vi "BCU参数读取-Auto.vi"(8 "CAN端口":u16(ring), 9 "设备索引号":u16(ring), 10 "CAN卡类型":u32(ring)=21, 11 "Myindex":dbl=1.0) -> (3 "成功":bool)   [LabVIEW 2013] (continued)
              n1586 = call <vilib>:"Unset Busy.vi"() -> ()  [unwired: 2 in, 10 out]
            }
          }
        }
        frame "模块软件版本读取" {
          n1587 = local read "从板板号"() -> (w2581:u8)
          n1588 = local read "模块软件版本"() -> (w2582:T1)
          n1589 = case shown="\"全部读取\"" w2582 {
            selector: w2582 -> [w2583 w2627]
            tunnel: w2581 -> [_ w2626]
            frame "BCUMCAL", Default {
              n1590 = stacked-sequence {
                seq-local: [_ _ w2609 _] -> [_ _ _ w2616]
                tunnel: w2583 -> [_ w2589 _ w2617]
                frame #0 {
                  w2588 = FALSE ("写?")
                  n1591 = call <vilib>:"Set Busy.vi"("disable click? (T)"=FALSE) -> ()  [unwired: 3 in, 8 out]
                  n1592 = local write "写?"(w2588) -> ()
                  n1593 = global write "EV05全局变量1.vi" "流控帧 2"(TRUE ("流控帧 2")) -> ()
                  n1594 = global write "EV05全局变量1.vi" "写入超时"(w2588) -> ()
                  n1595 = local write "控制1"(TRUE ("控制1")) -> ()
                  n1596 = local write "消除"(TRUE ("消除")) -> ()
                }
                frame #1 {
                  n1597 = Quotient & Remainder(x=w2589, y=256) -> (x-y*floor(x/y)=w2590:i32, floor(x/y)=w2591:i32)
                  n1598 = Build Array(w2591, w2590, u8 0 ("板号")) -> (w2594:i32[])
                  n1599 = local read "设备索引号"() -> (w2596:u16)
                  n1600 = local read "CAN卡类型"() -> (w2597:u32)
                  n1601 = local read "CAN端口"() -> (w2595:u16)
                  n1602 = stacked-sequence {
                    tunnel: w2597 -> [w2600 w2608]
                    tunnel: w2596 -> [w2599 w2607]
                    tunnel: w2595 -> [w2598 w2606]
                    tunnel: w2594 -> [_ w2605]
                    frame #0 {
                      n1603 = dll-call lib="PTH1abs FBluewave New EnergySVN_WorkAutoTest_TestStandtrunkAutoTest_TestStandDriverZlgCanBHN01è¯»ååæ°data\nkerneldlls\nusbcan.dll" fn="VCI_ClearBuffer"("DeviceType"=w2600, "DeviceInd"=w2599, "CANInd"=w2598) -> (error out=w2601:errorcluster)  [unwired: 4 in, 4 out]
                      n1604 = call <vilib>:"Clear Errors.vi"("error in (no error)"=w2601) -> ()  [unwired: 6 in, 1 out]
                    }
                    frame #1 {
                      w2604 = u8 137 ("命令")
                      w2602 = u32 3 ("命令序号")
                      n1605 = local read "从板板号"() -> (w2603:u8)
                      n1606 = local write "命令"(w2604) -> ()
                      n1607 = call "多帧发送机制(EV05).vi"("can卡类型"=w2608, "设备索引号"=w2607, "CAN端口"=w2606, "命令"=w2604, "板号"=w2603, "命令序号"=w2602, "输入数据"=w2605) -> ()  [unwired: 2 in, 11 out]
                      n1608 = local write "命令序号"(w2602) -> ()
                    }
                  }
                }
                frame #2 {
                  n1609 = while {
                    tunnel: [w2610] -> w2609
                    i -> [w2615]
                    stop <- w2611 stop-if-true
                    n1610 = global read "EV05全局变量1.vi" "写入超时"() -> (w2610:bool)
                    n1611 = Greater Or Equal?(x=w2615, y=25) -> (x >= y?=w2612:bool)
                    n1612 = Or(x=w2610, y=w2612) -> (x .or. y?=w2611:bool)
                    n1613 = Wait Until Next ms Multiple(millisecond multiple=u32 100 ("毫秒倍数")) -> ()  [unwired: 1 out]
                  }
                }
                frame #3 {
                  n1614 = call <vilib>:"Unset Busy.vi"() -> ()  [unwired: 2 in, 10 out]
                  n1615 = case shown="假" w2616 {
                    tunnel: w2617 -> [w2619 _]
                    frame False {
                      n1616 = Number To Decimal String(number=w2619) -> (decimal integer string=w2620:string)  [unwired: 1 out]
                      n1617 = control-ref of="结果"() -> (w2621:refnum<vi>)
                      n1618 = Concatenate Strings("模块" ("字符串"), w2620, "     读取失败" ("字符串")) -> (w2624:string)
                      n1619 = Build Array(w2624) -> (w2623:string[])
                      n1620 = call "表格编辑(版本读取).vi"("新元素/子数组"=w2623, "活动单元格:单元格背景色"=u32 16740749, "MCListbox引用句柄"=w2621) -> ()  [unwired: 9 out]
                    }
                    frame True {
                    }
                  }
                }
              }
            }
            frame "全部读取" {
              n1621 = stacked-sequence {
                seq-local: [w2628 _] -> [_ w2666]
                tunnel: w2627 -> [_ w2668]
                tunnel: w2626 -> [w2629 w2667]
                frame #0 {
                  n1622 = stacked-sequence {
                    tunnel: w2629 -> [_ w2638 _]
                    tunnel: [_ _ w2658] -> w2628
                    frame #0 {
                      w2634 = FALSE ("写?")
                      n1623 = control-ref of="模块软件版本 2"() -> (w2632:refnum<vi>)
                      n1624 = call <vilib>:"Set Busy.vi"("disable click? (T)"=FALSE) -> ()  [unwired: 3 in, 8 out]
                      n1625 = local write "写?"(w2634) -> ()
                      n1626 = property class="MCListbox (严格)"(reference=w2632, "ItemNames"=string[][] []) -> ()  [unwired: 1 in, 2 out]
                      n1627 = global write "EV05全局变量1.vi" "写入超时"(w2634) -> ()
                      n1628 = local write "消除"(TRUE ("消除")) -> ()
                      n1629 = global write "EV05全局变量1.vi" "流控帧 2"(TRUE ("流控帧 2")) -> ()
                      n1630 = local write "控制1"(TRUE ("控制1")) -> ()
                      n1631 = local write "MODEL号"(u8[] [] ("MODEL号")) -> ()
                    }
                    frame #1 {
                      n1632 = local read "设备索引号"() -> (w2640:u16)
                      n1633 = local read "CAN卡类型"() -> (w2641:u32)
                      n1634 = local read "CAN端口"() -> (w2639:u16)
                      n1635 = stacked-sequence {
                        tunnel: w2641 -> [w2644 w2657]
                        tunnel: w2640 -> [w2643 w2656]
                        tunnel: w2639 -> [w2642 w2655]
                        tunnel: w2638 -> [_ w2647]
                        frame #0 {
                          n1636 = dll-call lib="PTH1abs FBluewave New EnergySVN_WorkAutoTest_TestStandtrunkAutoTest_TestStandDriverZlgCanBHN01è¯»ååæ°data\nkerneldlls\nusbcan.dll" fn="VCI_ClearBuffer"("DeviceType"=w2644, "DeviceInd"=w2643, "CANInd"=w2642) -> (error out=w2645:errorcluster)  [unwired: 4 in, 4 out]
                          n1637 = call <vilib>:"Clear Errors.vi"("error in (no error)"=w2645) -> ()  [unwired: 6 in, 1 out]
                        }
                        frame #1 {
                          w2653 = u8 137 ("命令")
                          w2651 = u32 3 ("命令序号")
                          n1638 = Quotient & Remainder(x=u8 0 ("板号"), y=256) -> (x-y*floor(x/y)=w2648:i32, floor(x/y)=w2649:i32)
                          n1639 = local write "命令"(w2653) -> ()
                          n1640 = Build Array(w2649, w2648, u8 0 ("板号")) -> (w2654:i32[])
                          n1641 = call "多帧发送机制(EV05).vi"("can卡类型"=w2657, "设备索引号"=w2656, "CAN端口"=w2655, "命令"=w2653, "板号"=w2647, "命令序号"=w2651, "输入数据"=w2654) -> ()  [unwired: 2 in, 11 out]
                          n1642 = local write "命令序号"(w2651) -> ()
                        }
                      }
                    }
                    frame #2 {
                      n1643 = while {
                        tunnel: [w2660] -> w2658
                        i -> [w2664]
                        stop <- w2661 stop-if-true
                        n1644 = local read "强制停止版本读取"() -> (w2659:bool)
                        n1645 = global read "EV05全局变量1.vi" "写入超时"() -> (w2660:bool)
                        n1646 = Greater Or Equal?(x=w2664, y=35) -> (x >= y?=w2662:bool)
                        n1647 = Compound Arithmetic op=OR(w2659, w2660, w2662) -> (w2661:bool)
                        n1648 = Wait Until Next ms Multiple(millisecond multiple=u32 100 ("毫秒倍数")) -> ()  [unwired: 1 out]
                      }
                    }
                  }
                }
                frame #1 {
                  n1649 = case shown="真" w2666 {
                    tunnel: w2668 -> [_ w2678]
                    tunnel: w2667 -> [_ w2677]
                    frame False {
                      n1650 = control-ref of="结果"() -> (w2670:refnum<vi>)
                      n1651 = Concatenate Strings("模块编号" ("字符串"), "读取失败" ("字符串")) -> (w2673:string)
                      n1652 = Build Array(w2673) -> (w2672:string[])
                      n1653 = call "表格编辑(版本读取).vi"("新元素/子数组"=w2672, "活动单元格:单元格背景色"=u32 16740749, "MCListbox引用句柄"=w2670) -> ()  [unwired: 9 out]
                      n1654 = call <vilib>:"Unset Busy.vi"() -> ()  [unwired: 11 in, 1 out]
                    }
                    frame True {
                      n1655 = local read "MODEL号"() -> (w2676:u8[])
                      n1656 = Array Size(array=w2676) -> (size(s)=w2675:i32)
                      n1657 = for {
                        tunnel: w2678 -> [_]
                        tunnel: w2677 -> [w2681]
                        tunnel: w2676 -> [w2680] mode=indexing
                        tunnel: w2675 -> [w2679]
                        i -> [w2683]
                        n1658 = Increment(x=w2683) -> (x+1=w2682:i32)
                        n1659 = stacked-sequence {
                          seq-local: [_ _ _ w2710 _ _] -> [_ _ _ _ w2719 _]
                          seq-local: [_ w2689 _ _ _ _] -> [_ _ _ _ w2718 _]
                          tunnel: w2682 -> [_ _ _ _ _ w2730]
                          tunnel: w2680 -> [_ w2689 _ _ _ _]
                          tunnel: w2681 -> [_ w2690 _ _ _ _]
                          tunnel: w2679 -> [_ _ _ _ _ w2728]
                          frame #0 {
                            w2685 = FALSE ("写?")
                            n1660 = call <vilib>:"Set Busy.vi"("disable click? (T)"=FALSE) -> ()  [unwired: 3 in, 8 out]
                            n1661 = local write "写?"(w2685) -> ()
                            n1662 = global write "EV05全局变量1.vi" "写入超时"(w2685) -> ()
                            n1663 = global write "EV05全局变量1.vi" "流控帧 2"(TRUE ("流控帧 2")) -> ()
                            n1664 = local write "控制1"(TRUE ("控制1")) -> ()
                            n1665 = local write "消除"(TRUE ("消除")) -> ()
                          }
                          frame #1 {
                            n1666 = local read "设备索引号"() -> (w2692:u16)
                            n1667 = local read "CAN卡类型"() -> (w2693:u32)
                            n1668 = local read "CAN端口"() -> (w2691:u16)
                            n1669 = stacked-sequence {
                              tunnel: w2693 -> [w2696 w2709]
                              tunnel: w2692 -> [w2695 w2708]
                              tunnel: w2691 -> [w2694 w2707]
                              tunnel: w2690 -> [_ w2699]
                              tunnel: w2689 -> [_ w2698]
                              frame #0 {
                                n1670 = dll-call lib="PTH1abs FBluewave New EnergySVN_WorkAutoTest_TestStandtrunkAutoTest_TestStandDriverZlgCanBHN01è¯»ååæ°data\nkerneldlls\nusbcan.dll" fn="VCI_ClearBuffer"("DeviceType"=w2696, "DeviceInd"=w2695, "CANInd"=w2694) -> (error out=w2697:errorcluster)  [unwired: 4 in, 4 out]
                                n1671 = call <vilib>:"Clear Errors.vi"("error in (no error)"=w2697) -> ()  [unwired: 6 in, 1 out]
                              }
                              frame #1 {
                                w2705 = u8 137 ("命令")
                                w2703 = u32 3 ("命令序号")
                                n1672 = Quotient & Remainder(x=w2698, y=256) -> (x-y*floor(x/y)=w2700:i32, floor(x/y)=w2701:i32)
                                n1673 = local write "命令"(w2705) -> ()
                                n1674 = Build Array(w2701, w2700, u8 0 ("板号")) -> (w2706:i32[])
                                n1675 = call "多帧发送机制(EV05).vi"("can卡类型"=w2709, "设备索引号"=w2708, "CAN端口"=w2707, "命令"=w2705, "板号"=w2699, "命令序号"=w2703, "输入数据"=w2706) -> ()  [unwired: 2 in, 11 out]
                                n1676 = local write "命令序号"(w2703) -> ()
                              }
                            }
                          }
                          frame #2 {
                          }
                          frame #3 {
                            n1677 = while {
                              tunnel: [w2712] -> w2710
                              i -> [w2716]
                              stop <- w2713 stop-if-true
                              n1678 = local read "强制停止版本读取"() -> (w2711:bool)
                              n1679 = global read "EV05全局变量1.vi" "写入超时"() -> (w2712:bool)
                              n1680 = Greater Or Equal?(x=w2716, y=25) -> (x >= y?=w2714:bool)
                              n1681 = Compound Arithmetic op=OR(w2711, w2712, w2714) -> (w2713:bool)
                              n1682 = Wait Until Next ms Multiple(millisecond multiple=u32 100 ("毫秒倍数")) -> ()  [unwired: 1 out]
                            }
                          }
                          frame #4 {
                            n1683 = call <vilib>:"Unset Busy.vi"() -> ()  [unwired: 11 in, 1 out]
                            n1684 = case shown="假" w2719 {
                              tunnel: w2718 -> [w2721 _]
                              frame False {
                                n1685 = control-ref of="结果"() -> (w2723:refnum<vi>)
                                n1686 = Number To Decimal String(number=w2721) -> (decimal integer string=w2722:string)  [unwired: 1 out]
                                n1687 = Concatenate Strings("模块" ("字符串"), w2722, "     读取失败" ("字符串")) -> (w2726:string)
                                n1688 = Build Array(w2726) -> (w2725:string[])
                                n1689 = call "表格编辑(版本读取).vi"("新元素/子数组"=w2725, "活动单元格:单元格背景色"=u32 16740749, "MCListbox引用句柄"=w2723) -> ()  [unwired: 9 out]
                              }
                              frame True {
                              }
                            }
                          }
                          frame #5 {
                            n1690 = Equal?(x=w2728, y=w2730) -> (x = y?=w2729:bool)
                            n1691 = case shown="真" w2729 {
                              frame False {
                              }
                              frame True {
                                n1692 = control-ref of="模块软件版本 2"() -> (w2741:refnum<vi>)
                                n1693 = local read "模块版本名称"() -> (w2740:string[][])
                                n1694 = local read "模块版本值"() -> (w2736:string[][])
                                n1695 = control-ref of="结果"() -> (w2748:refnum<vi>)
                                n1696 = property class="MCListbox (严格)"(reference=w2741) -> ("ItemNames"=w2744:string[][])  [unwired: 1 in, 2 out]
                                n1697 = local read "从板板号"() -> (w2731:u8)
                                n1698 = Concatenate Strings("模块版本读取完成" ("字符串")) -> (w2751:string)
                                n1699 = Build Array(w2751) -> (w2750:string[])
                                n1700 = call "表格编辑(版本读取).vi"("新元素/子数组"=w2750, "活动单元格:单元格背景色"=u32 21937, "MCListbox引用句柄"=w2748) -> ()  [unwired: 9 out]
                                n1701 = Transpose 2D Array(2D array=w2744) -> (transposed array=w2745:string[][])
                                n1702 = local write "强制停止版本读取"(FALSE ("强制停止 2")) -> ()
                                n1703 = local read "模块个数"() -> (w2734:u8[])
                                n1704 = Index Array(array=w2745, index (row) #1=0 ("索引 (行)"), index (row) #2=1 ("索引 (行)")) -> (element #1=w2735:string[], element #2=w2737:string[])  [unwired: 2 in]
                                n1705 = Replace Array Subset(array=w2740, new element=w2735, index (row)=w2731) -> (w2739:string[][])  [unwired: 1 in]
                                n1706 = Replace Array Subset(array=w2736, new element=w2737, index (row)=w2731) -> (w2738:string[][])  [unwired: 1 in]
                                n1707 = local write "模块版本名称"(w2739) -> ()
                                n1708 = local write "模块版本值"(w2738) -> ()
                                n1709 = Array Size(array=w2735) -> (size(s)=w2732:i32)
                                n1710 = Replace Array Subset(array=w2734, new element=w2732, index=w2731) -> (w2733:u8[])
                                n1711 = local write "模块个数"(w2733) -> ()
                              }
                            }
                          }
                        }
                      }
                    }
                  }
                }
              }
            }
          }
        }
        frame "硬件版本读取" {
          n1712 = stacked-sequence {
            seq-local: [_ _ w2759 _] -> [_ _ _ w2766]
            frame #0 {
              w2755 = u8 137 ("命令")
              w2754 = u32 4 ("命令序号")
              n1713 = local read "设备索引号"() -> (w2757:u16)
              n1714 = local read "CAN卡类型"() -> (w2758:u32)
              n1715 = local read "CAN端口"() -> (w2756:u16)
              n1716 = local read "从板板号"() -> (w2752:u8)
              n1717 = local write "命令"(w2755) -> ()
              n1718 = call "多帧发送机制(EV05).vi"("can卡类型"=w2758, "设备索引号"=w2757, "CAN端口"=w2756, "命令"=w2755, "板号"=w2752, "命令序号"=w2754, "输入数据"=dbl[] [0.0]) -> ()  [unwired: 2 in, 11 out]
              n1719 = local write "命令序号"(w2754) -> ()
            }
            frame #1 {
            }
            frame #2 {
              n1720 = while {
                tunnel: [w2760] -> w2759
                i -> [w2765]
                stop <- w2761 stop-if-true
                n1721 = global read "EV05全局变量1.vi" "写入超时"() -> (w2760:bool)
                n1722 = Greater Or Equal?(x=w2765, y=25) -> (x >= y?=w2762:bool)
                n1723 = Or(x=w2760, y=w2762) -> (x .or. y?=w2761:bool)
                n1724 = Wait Until Next ms Multiple(millisecond multiple=u32 100 ("毫秒倍数")) -> ()  [unwired: 1 out]
              }
            }
            frame #3 {
              n1725 = case shown="假" w2766 {
                frame False {
                  n1726 = control-ref of="结果"() -> (w2768:refnum<vi>)
                  n1727 = Concatenate Strings("硬件版本" ("字符串"), "     读取失败" ("字符串")) -> (w2771:string)
                  n1728 = Build Array(w2771) -> (w2770:string[])
                  n1729 = call "表格编辑(版本读取).vi"("新元素/子数组"=w2770, "活动单元格:单元格背景色"=u32 16740749, "MCListbox引用句柄"=w2768) -> ()  [unwired: 9 out]
                }
                frame True {
                }
              }
              n1730 = call <vilib>:"Unset Busy.vi"() -> ()  [unwired: 2 in, 10 out]
            }
          }
        }
        frame "写配置文件" {
          n1731 = disable-structure shown="启用" {
            frame Enabled {
              n1732 = local read "主从选择"() -> (w2780:enum32{"主板", "从板"})
              n1733 = case shown="\"主板\", 默认" w2780 {
                tunnel: [w2799 w2990] -> w2783
                tunnel: ["M0" w2996] -> w2781
                frame "主板", Default {
                  n1734 = stacked-sequence {
                    seq-local: [w2813 _ _ _ _ _ _] -> [_ w2843 _ _ _ _ _]
                    seq-local: [string[] ["电池额定容量", "电池实际容量", "SOC", "SOH", "车牌号", "配置文件版本", "产品编号", "系统时钟"] _ _ _ _ _ _] -> [_ w2838 _ _ _ _ _]
                    seq-local: [_ _ _ _ string[] ["风机开启温度", "风机关闭温度", "加热开启温度", "加热关闭温度", "风机开启温差", "风机关闭温差", "加热关闭温差"] _ _] -> [_ _ _ _ _ w2942 _]
                    seq-local: [_ _ _ _ w2923 _ _] -> [_ _ _ _ _ w2940 _]
                    tunnel: [w2814 _ _ _ _ _ _] -> w2801
                    tunnel: [_ w2837 _ _ _ _ _] -> w2798
                    tunnel: [_ _ w2868 _ _ _ _] -> w2797
                    tunnel: [_ _ _ w2895 _ _ _] -> w2796
                    tunnel: [_ _ _ _ _ w2943 _] -> w2795
                    tunnel: [_ _ _ _ _ _ w2960] -> w2794
                    frame #0 {
                      w2805 = string[] ["", "", "", "", "", "", "", "", "", "", "  ", "", "", "", "", "", "", "", "", "", "  "]
                      n1735 = control-ref of="项目信息"() -> (w2833:refnum<vi>)
                      n1736 = property class="Tbl (严格)"(reference=w2833) -> ("Value"=w2809:string[][])  [unwired: 1 in, 2 out]
                      n1737 = control-ref of="项目信息2"() -> (w2827:refnum<vi>)
                      n1738 = Index Array(array=w2809, index (col)=0 ("禁用的索引 (列)")) -> (element=w2810:string[])  [unwired: 1 in]
                      n1739 = property class="Clust (严格)"(reference=w2827) -> ("Value"=w2826:T9)  [unwired: 1 in, 2 out]
                      n1740 = Index Array(array=w2809, index (col)=1 ("禁用的索引 (列)")) -> (element=w2808:string[])  [unwired: 1 in]
                      n1741 = local read "从板个数"() -> (w2832:dbl)
                      n1742 = Number To Decimal String(number=w2832) -> (decimal integer string=w2831:string)  [unwired: 1 out]
                      n1743 = Insert Into Array(array=w2810, new element=w2805) -> (w2807:string[])  [unwired: 1 in]
                      n1744 = Insert Into Array(array=w2808, new element=w2805) -> (w2806:string[])  [unwired: 1 in]
                      n1745 = Unbundle(w2826) -> ("电池额定容量(A)"=w2825:dbl, "电池实际容量(A)"=w2824:dbl, "车架(牌)号"=w2822:string, "配置文件版本"=w2821:string, "SOH(%)"=w2816:dbl, "SOC(%)"=w2815:dbl, "产品编号"=w2820:string, "系统时钟"=w2819:string)  [unwired: 1 out]
                      n1746 = Build Array("从板个数" ("元素"), w2831) -> (w2828:string[])
                      n1747 = Build Array(w2807, w2806) -> (w2803:string[][])
                      n1748 = Transpose 2D Array(2D array=w2803) -> (transposed array=w2802:string[][])
                      n1749 = Build Array(w2825, w2824, w2815, w2816) -> (w2823:dbl[])
                      n1750 = Build Array(w2822, w2821, w2820, w2819) -> (w2817:string[])
                      n1751 = for {
                        tunnel: w2823 -> [w2835] mode=indexing
                        tunnel: [w2834] -> w2818 mode=indexing
                        n1752 = Format Into String(format string="%#f" ("格式字符串"), w2835) -> (resulting string=w2834:string)  [unwired: 2 in, 1 out]
                      }
                      n1753 = Insert Into Array(array=w2802, index (row)=0 ("索引 (行)"), new element=w2828) -> (w2814:string[][])  [unwired: 1 in]
                      n1754 = Insert Into Array(array=w2818, new element=w2817) -> (w2813:string[])  [unwired: 1 in]
                    }
                    frame #1 {
                      n1755 = control-ref of="一级故障"() -> (w2864:refnum<vi>)
                      n1756 = property class="Clust (严格)"(reference=w2864) -> ("Value"=w2863:T10)  [unwired: 1 in, 2 out]
                      n1757 = Unbundle(w2863) -> ("总电压过高"=w2862:dbl, "整组电压不均衡"=w2857:dbl, "SOC过高"=w2850:dbl, "单体电压过高"=w2853:dbl, "总电压过低"=w2861:dbl, "温度过高"=w2860:dbl, "温度过低"=w2859:dbl, "单组电压不均衡"=w2858:dbl, "整组温度不均衡"=w2855:dbl, "单组温度不均衡"=w2856:dbl, "单体电压过低"=w2854:dbl, "充电电流过高"=w2852:dbl, "放电电流过高"=w2851:dbl, "SOC过低"=w2849:dbl, "内阻过大"=w2848:dbl, "极柱温度过高"=w2847:dbl, "SOH过低"=w2846:dbl)
                      n1758 = Build Array(w2862, w2861, w2860, w2859, w2858, w2857, w2856, w2855, w2853, w2854, w2852, w2851, w2850, w2849, w2848, w2847, w2846) -> (w2845:dbl[])
                      n1759 = for {
                        tunnel: w2845 -> [w2866] mode=indexing
                        tunnel: [w2865] -> w2842 mode=indexing
                        n1760 = Format Into String(format string="%#f" ("格式字符串"), w2866) -> (resulting string=w2865:string)  [unwired: 2 in, 1 out]
                      }
                      n1761 = Insert Into Array(array=w2843, new element=w2842) -> (w2841:string[])  [unwired: 1 in]
                      n1762 = Insert Into Array(array=w2838, new element=string[] ["总电压过高一级", "总电压过低一级", "温度过高一级", "温度过低一级", "单组电压不均衡一级", "整组电压不均衡一级", "单组温度不均衡一级", "整组温度不均衡一级", "单体电压过高一级", "单体电压过低一级", "充电电流过高一级", "放电电流过高一级", "SOC过高一级", "SOC过低一级", "内阻过大一级", "极柱温度过高一级", "SOH过低一级"]) -> (w2840:string[])  [unwired: 1 in]
                      n1763 = Build Array(w2840, w2841) -> (w2839:string[][])
                      n1764 = Transpose 2D Array(2D array=w2839) -> (transposed array=w2837:string[][])
                    }
                    frame #2 {
                      n1765 = control-ref of="一级故障 2"() -> (w2869:refnum<vi>)
                      n1766 = property class="Clust (严格)"(reference=w2869) -> ("Value"=w2891:T10)  [unwired: 1 in, 2 out]
                      n1767 = Unbundle(w2891) -> ("总电压过高"=w2890:dbl, "整组电压不均衡"=w2885:dbl, "SOC过高"=w2878:dbl, "单体电压过高"=w2881:dbl, "总电压过低"=w2889:dbl, "温度过高"=w2888:dbl, "温度过低"=w2887:dbl, "单组电压不均衡"=w2886:dbl, "整组温度不均衡"=w2883:dbl, "单组温度不均衡"=w2884:dbl, "单体电压过低"=w2882:dbl, "充电电流过高"=w2880:dbl, "放电电流过高"=w2879:dbl, "SOC过低"=w2877:dbl, "内阻过大"=w2876:dbl, "极柱温度过高"=w2875:dbl, "SOH过低"=w2874:dbl)
                      n1768 = Build Array(w2890, w2889, w2888, w2887, w2886, w2885, w2884, w2883, w2881, w2882, w2880, w2879, w2878, w2877, w2876, w2875, w2874) -> (w2873:dbl[])
                      n1769 = for {
                        tunnel: w2873 -> [w2893] mode=indexing
                        tunnel: [w2892] -> w2872 mode=indexing
                        n1770 = Format Into String(format string="%#f" ("格式字符串"), w2893) -> (resulting string=w2892:string)  [unwired: 2 in, 1 out]
                      }
                      n1771 = Build Array(string[] ["总电压过高二级", "总电压过低二级", "温度过高二级", "温度过低二级", "单组电压不均衡二级", "整组电压不均衡二级", "单组温度不均衡二级", "整组温度不均衡二级", "单体电压过高二级", "单体电压过低二级", "充电电流过高二级", "放电电流过高二级", "SOC过高二级", "SOC过低二级", "内阻过大二级", "极柱温度过高二级", "SOH过低二级"], w2872) -> (w2870:string[][])
                      n1772 = Transpose 2D Array(2D array=w2870) -> (transposed array=w2868:string[][])
                    }
                    frame #3 {
                      n1773 = control-ref of="一级故障 3"() -> (w2896:refnum<vi>)
                      n1774 = property class="Clust (严格)"(reference=w2896) -> ("Value"=w2918:T10)  [unwired: 1 in, 2 out]
                      n1775 = Unbundle(w2918) -> ("总电压过高"=w2917:dbl, "整组电压不均衡"=w2912:dbl, "SOC过高"=w2905:dbl, "单体电压过高"=w2908:dbl, "总电压过低"=w2916:dbl, "温度过高"=w2915:dbl, "温度过低"=w2914:dbl, "单组电压不均衡"=w2913:dbl, "整组温度不均衡"=w2910:dbl, "单组温度不均衡"=w2911:dbl, "单体电压过低"=w2909:dbl, "充电电流过高"=w2907:dbl, "放电电流过高"=w2906:dbl, "SOC过低"=w2904:dbl, "内阻过大"=w2903:dbl, "极柱温度过高"=w2902:dbl, "SOH过低"=w2901:dbl)
                      n1776 = Build Array(w2917, w2916, w2915, w2914, w2913, w2912, w2911, w2910, w2908, w2909, w2907, w2906, w2905, w2904, w2903, w2902, w2901) -> (w2900:dbl[])
                      n1777 = for {
                        tunnel: w2900 -> [w2920] mode=indexing
                        tunnel: [w2919] -> w2899 mode=indexing
                        n1778 = Format Into String(format string="%#f" ("格式字符串"), w2920) -> (resulting string=w2919:string)  [unwired: 2 in, 1 out]
                      }
                      n1779 = Build Array(string[] ["总电压过高三级", "总电压过低三级", "温度过高三级", "温度过低三级", "单组电压不均衡三级", "整组电压不均衡三级", "单组温度不均衡三级", "整组温度不均衡三级", "单体电压过高三级", "单体电压过低三级", "充电电流过高三级", "放电电流过高三级", "SOC过高三级", "SOC过低三级", "内阻过大三级", "极柱温度过高三级", "SOH过低三级"], w2899) -> (w2897:string[][])
                      n1780 = Transpose 2D Array(2D array=w2897) -> (transposed array=w2895:string[][])
                    }
                    frame #4 {
                      n1781 = control-ref of="加热控制参数"() -> (w2933:refnum<vi>)
                      n1782 = property class="Clust (严格)"(reference=w2933) -> ("Value"=w2932:T11)  [unwired: 1 in, 2 out]
                      n1783 = Unbundle(w2932) -> ("风机开启温度"=w2931:dbl, "风机关闭温度"=w2930:dbl, "加热开启温度"=w2929:dbl, "加热关闭温度"=w2928:dbl, "风机开启温差"=w2927:dbl, "风机关闭温差"=w2926:dbl, "加热关闭温差"=w2922:dbl)
                      n1784 = Build Array(w2931, w2930, w2929, w2928, w2927, w2926, w2922) -> (w2925:dbl[])
                      n1785 = for {
                        tunnel: w2925 -> [w2935] mode=indexing
                        tunnel: [w2934] -> w2923 mode=indexing
                        n1786 = Format Into String(format string="%#f" ("格式字符串"), w2935) -> (resulting string=w2934:string)  [unwired: 2 in, 1 out]
                      }
                    }
                    frame #5 {
                      n1787 = control-ref of="充电控制参数"() -> (w2953:refnum<vi>)
                      n1788 = property class="Clust (严格)"(reference=w2953) -> ("Value"=w2955:T12)  [unwired: 1 in, 2 out]
                      n1789 = Unbundle(w2955) -> ("最大允许单体电压"=w2952:dbl, "最大允许总电压"=w2951:dbl, "最小允许单体电压"=w2950:dbl, "最大允许充电电流"=w2949:dbl, "最小允许充电电流"=w2948:dbl, "最大允许充电温度"=w2947:dbl, "最小允许充电温度"=w2946:dbl, "电流步长"=w2945:dbl)
                      n1790 = Build Array(w2952, w2951, w2950, w2949, w2948, w2947, w2946, w2945) -> (w2954:dbl[])
                      n1791 = for {
                        tunnel: w2954 -> [w2957] mode=indexing
                        tunnel: [w2956] -> w2939 mode=indexing
                        n1792 = Format Into String(format string="%#f" ("格式字符串"), w2957) -> (resulting string=w2956:string)  [unwired: 2 in, 1 out]
                      }
                      n1793 = Insert Into Array(array=w2940, new element=w2939) -> (w2938:string[])  [unwired: 1 in]
                      n1794 = Insert Into Array(array=w2942, new element=string[] ["最大允许单体电压", "最大允许总电压", "最小允许单体电压", "最大允许充电电流", "最小允许充电电流", "最大允许充电温度", "最小允许充电温度", "电流步长"]) -> (w2937:string[])  [unwired: 1 in]
                      n1795 = Build Array(w2937, w2938) -> (w2944:string[][])
                      n1796 = Transpose 2D Array(2D array=w2944) -> (transposed array=w2943:string[][])
                    }
                    frame #6 {
                      n1797 = control-ref of="电池信息"() -> (w2981:refnum<vi>)
                      n1798 = property class="Clust (严格)"(reference=w2981) -> ("Value"=w2984:T13)  [unwired: 1 in, 2 out]
                      n1799 = Unbundle(w2984) -> ("电池串联"=w2980:dbl, "电池并联"=w2979:dbl, "累计放电总安时"=w2977:dbl, "电池包额定容量"=w2976:dbl, "电池包额定能量(kWh)"=w2975:dbl, "电池包额定总电压"=w2974:dbl, "累计充电总安时"=w2978:dbl, "电池充满次数"=w2973:dbl, "电池放空次数"=w2972:dbl, "电池充电次数"=w2971:dbl, "电池生产日期"=w2969:string, "电池厂家"=w2968:string, "电池类型"=w2967:string, "电池包组号"=w2966:string, "电池包产权标识"=w2965:string, "电池应用车型"=w2964:string, "实际容量"=w2959:dbl)
                      n1800 = Build Array(w2969, w2968, w2967, w2966, w2965, w2964) -> (w2963:string[])
                      n1801 = Build Array(w2980, w2979, w2978, w2977, w2976, w2975, w2974, w2973, w2972, w2971, w2959) -> (w2970:dbl[])
                      n1802 = for {
                        tunnel: w2970 -> [w2986] mode=indexing
                        tunnel: [w2985] -> w2962 mode=indexing
                        n1803 = Format Into String(format string="%#f" ("格式字符串"), w2986) -> (resulting string=w2985:string)  [unwired: 2 in, 1 out]
                      }
                      n1804 = Insert Into Array(array=w2963, new element=w2962) -> (w2961:string[])  [unwired: 1 in]
                      n1805 = call <vilib>:"Unset Busy.vi"() -> ()  [unwired: 2 in, 10 out]
                      n1806 = Build Array(string[] ["电池生产日期", "电池厂商", "电池类型", "电池包组号", "电池包产权标识", "电池包应用车型", "电池串联", "电池并联", "累计充电总安时", "累计放电总安时", "电池包额定容量", "电池包额定能量", "电池包额定总电压", "电池充满次数", "电池放空次数", "电池充电次数", "实际容量"], w2961) -> (w2982:string[][])
                      n1807 = Transpose 2D Array(2D array=w2982) -> (transposed array=w2960:string[][])
                    }
                  }
                  n1808 = Insert Into Array(array=w2801, index (col)=2 ("禁用的索引 (列)"), new element #1=w2798, new element #2=w2797, new element #3=w2796, new element #4=w2795, new element #5=w2794) -> (w2799:string[][])  [unwired: 1 in]
                }
                frame "从板" {
                  n1809 = local read "从板号"() -> (w2998:u8)
                  n1810 = Number To Decimal String(number=w2998) -> (decimal integer string=w2995:string)  [unwired: 1 out]
                  n1811 = Concatenate Strings("S", w2995) -> (w2996:string)
                  n1812 = Build Array("从板号" ("元素"), w2995) -> (w2993:string[])
                  n1813 = stacked-sequence {
                    seq-local: [string[] ["风机开启温度", "风机关闭温度", "加热开启温度", "加热关闭温度", "风机开启温差", "风机关闭温差", "加热关闭温差"] _ _ _ _ _] -> [_ _ _ w3067 _ _]
                    seq-local: [w3010 _ _ _ _ _] -> [_ _ _ w3063 _ _]
                    seq-local: [_ string[] ["电压过高一级", "电压过低一级", "温度过高一级", "温度过低一级", "电压不均衡一级", "温度不均衡一级", "SOC过低一级"] _ _ _ _] -> [_ _ _ w3066 _ _]
                    seq-local: [_ w3028 _ _ _ _] -> [_ _ _ w3062 _ _]
                    seq-local: [_ _ string[] ["电压过高二级", "电压过低二级", "温度过高二级", "温度过低二级", "电压不均衡二级", "温度不均衡二级", "SOC过低二级"] _ _ _] -> [_ _ _ w3065 _ _]
                    seq-local: [_ _ w3043 _ _ _] -> [_ _ _ w3061 _ _]
                    tunnel: w2993 -> [w3023 _ _ _ _ _]
                    tunnel: [w3012 _ _ _ _ _] -> w2991
                    tunnel: [_ _ _ w3068 _ _] -> w2989
                    tunnel: [_ _ _ _ w3106 _] -> w2988
                    tunnel: [_ _ _ _ _ w3142] -> _
                    frame #0 {
                      w3003 = string[] ["", "", "", "", "", "", "", "", "", "", "  "]
                      n1814 = control-ref of="项目信息 2"() -> (w3022:refnum<vi>)
                      n1815 = property class="Tbl (严格)"(reference=w3022) -> ("Value"=w3000:string[][])  [unwired: 1 in, 2 out]
                      n1816 = control-ref of="加热控制参数"() -> (w3014:refnum<vi>)
                      n1817 = property class="Clust (严格)"(reference=w3014) -> ("Value"=w3021:T11)  [unwired: 1 in, 2 out]
                      n1818 = Unbundle(w3021) -> ("风机开启温度"=w3020:dbl, "风机关闭温度"=w3019:dbl, "加热开启温度"=w3018:dbl, "加热关闭温度"=w3017:dbl, "风机开启温差"=w3016:dbl, "风机关闭温差"=w3015:dbl, "加热关闭温差"=w3009:dbl)
                      n1819 = Build Array(w3020, w3019, w3018, w3017, w3016, w3015, w3009) -> (w3013:dbl[])
                      n1820 = for {
                        tunnel: w3013 -> [w3026] mode=indexing
                        tunnel: [w3025] -> w3010 mode=indexing
                        n1821 = Format Into String(format string="%#f" ("格式字符串"), w3026) -> (resulting string=w3025:string)  [unwired: 2 in, 1 out]
                      }
                      n1822 = Index Array(array=w3000, index (col)=0 ("禁用的索引 (列)")) -> (element=w3007:string[])  [unwired: 1 in]
                      n1823 = Index Array(array=w3000, index (col)=1 ("禁用的索引 (列)")) -> (element=w3006:string[])  [unwired: 1 in]
                      n1824 = Insert Into Array(array=w3007, new element=w3003) -> (w3005:string[])  [unwired: 1 in]
                      n1825 = Insert Into Array(array=w3006, new element=w3003) -> (w3004:string[])  [unwired: 1 in]
                      n1826 = Build Array(w3005, w3004) -> (w3001:string[][])
                      n1827 = Transpose 2D Array(2D array=w3001) -> (transposed array=w2999:string[][])
                      n1828 = Insert Into Array(array=w2999, index (row)=0 ("索引 (行)"), new element=w3023) -> (w3012:string[][])  [unwired: 1 in]
                    }
                    frame #1 {
                      n1829 = control-ref of="一级故障(从板)"() -> (w3039:refnum<vi>)
                      n1830 = property class="Clust (严格)"(reference=w3039) -> ("Value"=w3038:T15)  [unwired: 1 in, 2 out]
                      n1831 = Unbundle(w3038) -> ("电压过高"=w3037:dbl, "电压过低"=w3036:dbl, "温度过高"=w3035:dbl, "温度过低"=w3034:dbl, "电压不均衡(V)"=w3033:dbl, "温度不均衡"=w3032:dbl, "SOC过低"=w3031:dbl)
                      n1832 = Build Array(w3037, w3036, w3035, w3034, w3033, w3032, w3031) -> (w3030:dbl[])
                      n1833 = for {
                        tunnel: w3030 -> [w3041] mode=indexing
                        tunnel: [w3040] -> w3028 mode=indexing
                        n1834 = Format Into String(format string="%#f" ("格式字符串"), w3041) -> (resulting string=w3040:string)  [unwired: 2 in, 1 out]
                      }
                    }
                    frame #2 {
                      n1835 = control-ref of="二级故障(从板)"() -> (w3045:refnum<vi>)
                      n1836 = property class="Clust (严格)"(reference=w3045) -> ("Value"=w3054:T15)  [unwired: 1 in, 2 out]
                      n1837 = Unbundle(w3054) -> ("电压过高"=w3053:dbl, "电压过低"=w3052:dbl, "温度过高"=w3051:dbl, "温度过低"=w3050:dbl, "电压不均衡(V)"=w3049:dbl, "温度不均衡"=w3048:dbl, "SOC过低"=w3047:dbl)
                      n1838 = Build Array(w3053, w3052, w3051, w3050, w3049, w3048, w3047) -> (w3046:dbl[])
                      n1839 = for {
                        tunnel: w3046 -> [w3056] mode=indexing
                        tunnel: [w3055] -> w3043 mode=indexing
                        n1840 = Format Into String(format string="%#f" ("格式字符串"), w3056) -> (resulting string=w3055:string)  [unwired: 2 in, 1 out]
                      }
                    }
                    frame #3 {
                      n1841 = control-ref of="三级故障(从板)"() -> (w3069:refnum<vi>)
                      n1842 = property class="Clust (严格)"(reference=w3069) -> ("Value"=w3079:T15)  [unwired: 1 in, 2 out]
                      n1843 = Unbundle(w3079) -> ("电压过高"=w3078:dbl, "电压过低"=w3077:dbl, "温度过高"=w3076:dbl, "温度过低"=w3075:dbl, "电压不均衡(V)"=w3074:dbl, "温度不均衡"=w3073:dbl, "SOC过低"=w3072:dbl)
                      n1844 = Build Array(w3078, w3077, w3076, w3075, w3074, w3073, w3072) -> (w3071:dbl[])
                      n1845 = for {
                        tunnel: w3071 -> [w3081] mode=indexing
                        tunnel: [w3080] -> w3060 mode=indexing
                        n1846 = Format Into String(format string="%#f" ("格式字符串"), w3081) -> (resulting string=w3080:string)  [unwired: 2 in, 1 out]
                      }
                      n1847 = Insert Into Array(array=w3067, new element #1=w3066, new element #2=w3065, new element #3=string[] ["电压过高三级", "电压过低三级", "温度过高三级", "温度过低三级", "电压不均衡三级", "温度不均衡三级", "SOC过低三级"]) -> (w3058:string[])  [unwired: 1 in]
                      n1848 = Insert Into Array(array=w3063, new element #1=w3062, new element #2=w3061, new element #3=w3060) -> (w3059:string[])  [unwired: 1 in]
                      n1849 = Build Array(w3058, w3059) -> (w3070:string[][])
                      n1850 = Transpose 2D Array(2D array=w3070) -> (transposed array=w3068:string[][])
                    }
                    frame #4 {
                      n1851 = control-ref of="快换(从板)"() -> (w3105:refnum<vi>)
                      n1852 = property class="Clust (严格)"(reference=w3105) -> ("Value"=w3118:T16)  [unwired: 1 in, 2 out]
                      n1853 = Unbundle(w3118) -> ("串联数"=w3117:dbl, "并联数"=w3116:dbl, "电池厂家"=w3115:dbl, "电池类型"=w3114:dbl, "额定能量"=w3113:dbl, "额定容量"=w3112:dbl, "实际容量"=w3111:dbl, "额定总压"=w3104:dbl, "产权标识"=w3103:dbl, "应用车型"=w3102:dbl, "电池包组号"=w3101:dbl, "SOC"=w3099:dbl, "充电总安时"=w3098:dbl, "放电总安时"=w3097:dbl, "放空次数"=w3096:dbl, "充满次数"=w3095:dbl, "充电次数"=w3094:dbl, "车牌号"=w3084:string, "生产日期"=w3083:string, "最大允许单体电压"=w3093:dbl, "最大允许总电压"=w3092:dbl, "最大允许温度"=w3091:dbl, "最小允许温度"=w3090:dbl, "最大允许充电电流"=w3089:dbl, "最小允许充电电流"=w3088:dbl, "最小允许单体电压"=w3087:dbl, "电流步长"=w3086:dbl, "电池包序号"=w3085:dbl)
                      n1854 = Build Array(w3117, w3116, w3115, w3114, w3113, w3112, w3111, w3104, w3103, w3102, w3101, w3099, w3098, w3097, w3096, w3095, w3094, w3093, w3092, w3091, w3090, w3089, w3088, w3087, w3086, w3085) -> (w3110:dbl[])
                      n1855 = for {
                        tunnel: w3110 -> [w3120] mode=indexing
                        tunnel: [w3119] -> w3108 mode=indexing
                        n1856 = Format Into String(format string="%#f" ("格式字符串"), w3120) -> (resulting string=w3119:string)  [unwired: 2 in, 1 out]
                      }
                      n1857 = Insert Into Array(array=w3108, new element #1=w3084, new element #2=w3083) -> (w3100:string[])  [unwired: 1 in]
                      n1858 = call <vilib>:"Unset Busy.vi"() -> ()  [unwired: 2 in, 10 out]
                      n1859 = Build Array(string[] ["电池串联数", "电池并联数", "电池厂家", "额定能量", "额定容量", "实际容量", "额定总压", "产权标识", "应用车型", "电池包组号", "SOC", "充电总安时", "放电总安时", "放空次数", "充满次数", "充电次数", "最大允许单体电压", "最大允许总电压", "最大允许温度", "最小允许温度", "最大允许充电电流", "最小允许充电电流", "最小允许单体电压", "电流步长", "电池包序号"], w3100) -> (w3109:string[][])
                      n1860 = Transpose 2D Array(2D array=w3109) -> (transposed array=w3106:string[][])
                    }
                    frame #5 {
                      n1861 = local read "均衡参数"() -> (w3141:T17)
                      n1862 = Unbundle(w3141) -> ("充电结束电压(90%)"=w3133:sgl, "充电结束电压(91%)"=w3132:sgl, "充电结束电压(92%)"=w3131:sgl, "充电结束电压(93%)"=w3130:sgl, "充电结束电压(94%)"=w3129:sgl, "均衡计算-电压高阀值1级"=w3140:sgl, "均衡计算-电压高阀值2级"=w3139:sgl, "均衡计算-电压低阀值1级"=w3138:sgl, "均衡计算-电压低阀值2级"=w3137:sgl, "均衡计算-最低电压阀值"=w3136:sgl, "均衡停止-最低电压阀值"=w3135:sgl, "均衡计算-电压极差阀值"=w3134:sgl, "充电结束电压(95%)"=w3128:sgl, "充电结束电压(96%)"=w3127:sgl, "充电结束电压(97%)"=w3126:sgl, "充电结束电压(98%)"=w3125:sgl, "充电结束电压(99%)"=w3124:sgl, "充电结束电压(100%)"=w3123:sgl)
                      n1863 = Build Array(w3140, w3139, w3138, w3137, w3136, w3135, w3134, w3133, w3132, w3131, w3130, w3129, w3128, w3127, w3126, w3125, w3124, w3123) -> (w3145:sgl[])
                      n1864 = for {
                        tunnel: w3145 -> [w3147] mode=indexing
                        tunnel: [w3146] -> w3122 mode=indexing
                        n1865 = Format Into String(format string="%#f" ("格式字符串"), w3147) -> (resulting string=w3146:string)  [unwired: 2 in, 1 out]
                      }
                      n1866 = call <vilib>:"Unset Busy.vi"() -> ()  [unwired: 2 in, 10 out]
                      n1867 = Build Array(string[] ["均衡计算-电压高阀值1级", "均衡计算-电压高阀值2级", "均衡计算-电压低阀值1级", "均衡计算-电压低阀值2级", "均衡计算-最低电压阀值", "均衡停止-最低电压阀值", "均衡计算-电压极差阀值", "充电结束电压(90%)", "充电结束电压(91%)", "充电结束电压(92%)", "充电结束电压(93%)", "充电结束电压(94%)", "充电结束电压(95%)", "充电结束电压(96%)", "充电结束电压(97%)", "充电结束电压(98%)", "充电结束电压(99%)", "充电结束电压(100%)"], w3122) -> (w3144:string[][])
                      n1868 = Transpose 2D Array(2D array=w3144) -> (transposed array=w3142:string[][])
                    }
                  }
                  n1869 = Insert Into Array(array=w2991, index (col)=2 ("禁用的索引 (列)"), new element #1=w2989, new element #2=w2988) -> (w2990:string[][])  [unwired: 1 in]
                }
              }
              n1870 = call "当前时间解析-8.6.vi"() -> ("名称格式时间"=w2782:string)  [unwired: 1 in, 18 out]
              n1871 = Concatenate Strings(w2782, w2781, ".txt" ("字符串")) -> (w2779:string)
              n1872 = call "自适应屏幕分辨率.vi"() -> ()  [unwired: 16 in]
              n1873 = call "文件对话框2"("prompt"="选择保存的路径", "default name"=w2779, "pattern (all files)"="*.txt") -> ("selected path"=w2777:path, "cancelled"=w2776:bool, "error out"=w2775:errorcluster)  [unwired: 9 in, 1 out]
              n1874 = call <vilib>:"Clear Errors.vi"("error in (no error)"=w2775) -> ()  [unwired: 6 in, 1 out]
              n1875 = case shown="假" w2776 {
                tunnel: w2783 -> [w2788 _]
                tunnel: w2777 -> [w2784 _]
                frame False {
                  n1876 = call-poly <vilib>:"Write To Spreadsheet File.vi"("append to file? (new file:F)"=FALSE, "2D data"=w2788, "file path (dialog if empty)"=w2784) -> ("new file path (Not A Path if cancelled)"=w2786:path)  [unwired: 3 in, 2 out]
                  n1877 = Path To String(path=w2786) -> (string=w2785:string)
                  n1878 = stacked-sequence {
                    tunnel: w2785 -> [w2791]
                    frame #0 {
                      n1879 = Concatenate Strings("保存完成,路径为:" ("字符串"), w2791) -> (w2792:string)
                      n1880 = One Button Dialog(message=w2792, button name ("OK")="是" ("按钮名称（“确定”）")) -> ()  [unwired: 1 out]
                    }
                  }
                }
                frame True {
                }
              }
            }
            frame Disabled {
              n1881 = stacked-sequence {
                seq-local: [w3162] -> [_]
                frame #0 {
                  n1882 = local read "项目信息"() -> (w3164:string[][])
                  n1883 = local read "项目信息2"() -> (w3161:T9)
                  n1884 = Array Subset(array=w3164, index (row)=0 ("索引"), index (col)=0 ("索引"), length (col)=2 ("索引")) -> (w3167:string[][])  [unwired: 1 in]
                  n1885 = local read "一级故障"() -> ()  [unwired: 1 out]
                  n1886 = local read "从板个数"() -> (w3162:dbl)
                  n1887 = Unbundle(w3161) -> ("电池额定容量(A)"=w3160:dbl, "电池实际容量(A)"=w3159:dbl, "车架(牌)号"=w3153:string, "配置文件版本"=w3152:string, "SOH(%)"=w3157:dbl, "SOC(%)"=w3158:dbl, "产品编号"=w3154:string)  [unwired: 2 out]
                  n1888 = Index Array(array=w3167, index (col) #1=1 ("禁用的索引 (列)"), index (col) #2=0 ("索引 (列)")) -> (element #1=w3151:string[], element #2=w3150:string[])  [unwired: 2 in]
                  n1889 = Build Array(w3160, w3159, w3158, w3157) -> (w3156:dbl[])
                  n1890 = Number To Decimal String(number=w3162) -> ()  [unwired: 1 in, 1 out]
                  n1891 = for {
                    tunnel: w3156 -> [w3172] mode=indexing
                    tunnel: [w3171] -> w3155 mode=indexing
                    n1892 = Format Into String(format string="%#f" ("格式字符串"), w3172) -> (resulting string=w3171:string)  [unwired: 2 in, 1 out]
                  }
                  n1893 = Insert Into Array(array=w3155, new element #1=w3154, new element #2=w3153, new element #3=w3152, new element #4=w3151) -> ()  [unwired: 1 in, 1 out]
                  n1894 = Insert Into Array(array=string[] ["电池额定容量", "电池实际容量", "SOC", "SOH", "产品编号", "车架(牌)号", "配置文件版本"], new element=w3150) -> ()  [unwired: 1 in, 1 out]
                }
              }
            }
          }
        }
        frame "读配置文件" {
        }
      }
    }
    frame Error {
    }
  }
  n1895 = while {
    tunnel: w26 -> [w3184]
    tunnel: w25 -> [w3183]
    tunnel: [w3182] -> w29
    tunnel: [w3181] -> w28
    tunnel: w21 -> [_]
    tunnel: w24 -> [w3173]
    stop <- w3180 stop-if-true
    n1896 = local read "停止"() -> (w3180:bool)
    n1897 = local read "设备索引号"() -> (w3177:u16)
    n1898 = local read "CAN卡类型"() -> (w3178:u32)
    n1899 = local read "CAN端口"() -> (w3176:u16)
    n1900 = call "receiver-8.6.vi"("错误输入（无错误）"=w3173, "CAN端口"=w3176, "设备索引号"=w3177, "CAN卡类型"=w3178) -> ("错误输出"=w3179:errorcluster, "输出簇"=w3175:T27, "接收成功"=w3174:bool)  [unwired: 3 out]
    n1901 = call <vilib>:"Clear Errors.vi"("error in (no error)"=w3179) -> ()  [unwired: 6 in, 1 out]
    n1902 = case shown="真" w3174 {
      tunnel: w3183 -> [w3185 w3191]
      tunnel: w3175 -> [_ w3190]
      tunnel: w3184 -> [w3186 w3189]
      tunnel: [w3186 w3188] -> w3182
      tunnel: [w3185 w3187] -> w3181
      frame False {
      }
      frame True {
        n1903 = Enqueue Element(queue=w3189, element=w3190, error in (no error)=w3191) -> (queue out=w3188:refnum<queue>, error out=w3187:errorcluster)  [unwired: 2 out]
      }
    }
  }
  n1904 = while {
    tunnel: w26 -> [w3199]
    tunnel: w25 -> [w3198]
    stop <- w3192 stop-if-true
    n1905 = local read "停止"() -> (w3192:bool)
    n1906 = local read "控制1"() -> (w3194:bool)
    n1907 = Dequeue Element(queue=w3199, timeout in ms (-1)=200 ("超时毫秒(-1)"), error in (no error)=w3198) -> (element=w3197:T3, error out=w3196:errorcluster)  [unwired: 2 out]
    n1908 = case shown="无错误" w3196 {
      tunnel: w3197 -> [w3204 _]
      tunnel: "写?" -> [w3201 _]
      tunnel: w3194 -> [w3200 _]
      frame No Error {
        n1909 = Unbundle(w3204) -> ("return type"=w3203:u32, "pReceive"=w3202:T28)
        n1910 = for {
          N: w3203 -> [_]
          tunnel: w3202 -> [w3208] mode=indexing
          tunnel: w3201 -> [w3206]
          tunnel: w3200 -> [w3205]
          n1911 = Unbundle By Name(w3208) -> ("ID"=w3209:u32)
          n1912 = call "ID解析.vi"("ID"=w3209) -> ("PDU(1)"=w3207:i32)  [unwired: 10 out]
          n1913 = case shown="18" w3207 {
            tunnel: w3208 -> [_ w3219]
            tunnel: w3206 -> [_ w3211]
            tunnel: w3205 -> [_ w3210]
            frame 0, Default {
            }
            frame 24 {
              n1914 = local read "主从选择"() -> (w3212:enum32{"主板", "从板"})
              n1915 = local read "设备索引号"() -> (w3215:u16)
              n1916 = local read "CAN卡类型"() -> (w3214:u32)
              n1917 = local read "CAN端口"() -> (w3216:u16)
              n1918 = disable-structure shown="禁用" {
                disable-tunnel: w3219 -> [w3222 _]
                frame Disabled {
                  n1919 = call "标定授权读取.vi"("VCI_Receive"=w3222) -> ()  [unwired: 1 out]
                }
                frame Enabled {
                }
              }
              n1920 = case shown="\"从板\"" w3212 {
                tunnel: [0 ("FUNC") w3221] -> w3213
                frame "主板", Default {
                }
                frame "从板" {
                  n1921 = local read "从板号"() -> (w3221:u8)
                }
              }
              n1922 = local read "面板选择"() -> (w3218:T7)
              n1923 = case shown="\"读写参数\", 默认" w3218 {
                tunnel: w3211 -> [w3229 _ _ _]
                tunnel: "命令" -> [w3230 w3334 w3589 w3729]
                tunnel: w3212 -> [w3239 _ w3597 w3737]
                tunnel: w3219 -> [_ _ _ _]
                tunnel: w3219 -> [w3235 w3335 w3591 w3731]
                tunnel: w3216 -> [w3234 w3336 w3592 w3732]
                tunnel: w3215 -> [w3233 w3337 w3593 w3733]
                tunnel: w3214 -> [w3232 w3338 w3594 w3734]
                tunnel: w3213 -> [w3231 _ w3590 w3730]
                tunnel: w3210 -> [w3225 _ _ _]
                frame "读写参数", Default {
                  n1924 = control-ref of="流控帧 2"() -> (w3223:refnum<vi>)
                  n1925 = control-ref of="流控帧"() -> (w3224:refnum<vi>)
                  n1926 = local read "命令序号"() -> (w3228:u8)
                  n1927 = call "多帧接收机制(EV05).vi"("can卡类型"=w3232, "设备索引号"=w3233, "CAN端口"=w3234, "VCI_Receive"=w3235, "命令"=w3230, "板号"=w3231, "流控帧"=w3224, "写?"=w3229, "流控帧2"=w3223, "命令序号"=w3228) -> ("错误信号"=w3226:bool, "错误代码"=w3238:i32, "输出数组"=w3237:u8[], "读错误代码"=w3227:u8[], "结束信号"=w3236:bool)  [unwired: 5 out]
                  n1928 = case shown="假" w3229 {
                    tunnel: w3236 -> [w3249 w3317]
                    tunnel: w3238 -> [w3248 w3316]
                    tunnel: w3228 -> [w3247 _]
                    tunnel: w3237 -> [w3246 _]
                    tunnel: w3230 -> [w3245 _]
                    tunnel: w3239 -> [w3243 w3315]
                    tunnel: w3227 -> [w3242 _]
                    tunnel: w3226 -> [w3241 _]
                    tunnel: w3225 -> [w3240 _]
                    frame False {
                      # "读参数"
                      n1929 = And(x=w3240, y=w3249) -> (x .and. y?=w3244:bool)
                      n1930 = case shown="真" w3244 {
                        tunnel: w3248 -> [_ w3260]
                        tunnel: w3247 -> [_ w3259]
                        tunnel: w3246 -> [_ w3258]
                        tunnel: w3245 -> [_ w3257]
                        tunnel: w3243 -> [_ w3253]
                        tunnel: w3242 -> [_ w3251]
                        tunnel: w3241 -> [_ w3252]
                        frame False {
                        }
                        frame True {
                          n1931 = case shown="假" w3252 {
                            tunnel: w3260 -> [w3272 _]
                            tunnel: w3259 -> [w3271 _]
                            tunnel: w3258 -> [w3270 _]
                            tunnel: w3257 -> [w3268 _]
                            tunnel: w3253 -> [w3264 _]
                            tunnel: w3251 -> [_ w3300]
                            frame False {
                              n1932 = case shown="\"主板\", 默认" w3264 {
                                tunnel: [w3274 _] -> w3267
                                tunnel: [_ w3288] -> w3266
                                tunnel: [w3273 _] -> w3263
                                frame "主板", Default {
                                n1933 = stacked-sequence {
                                tunnel: [_ w3287] -> w3274
                                tunnel: [w3275 _] -> w3273
                                frame #0 {
                                n1934 = control-ref of="一级故障"() -> (w3281:refnum<vi>)
                                n1935 = control-ref of="一级故障 2"() -> (w3283:refnum<vi>)
                                n1936 = control-ref of="一级故障 3"() -> (w3284:refnum<vi>)
                                n1937 = control-ref of="加热控制参数"() -> (w3285:refnum<vi>)
                                n1938 = control-ref of="充电控制参数"() -> (w3286:refnum<vi>)
                                n1939 = control-ref of="电池信息"() -> (w3279:refnum<vi>)
                                n1940 = control-ref of="项目信息"() -> (w3282:refnum<vi>)
                                n1941 = control-ref of="项目信息2"() -> (w3280:refnum<vi>)
                                n1942 = control-ref of="高压参数"() -> (w3278:refnum<vi>)
                                n1943 = local read "主板数据"() -> (w3277:T4)
                                n1944 = Bundle(cluster=w3277, "项目信息"=w3282, "一级故障 4"=w3280, "一级故障"=w3281, "一级故障 2"=w3283, "一级故障 3"=w3284, "加热控制参数"=w3285, "充电控制参数"=w3286, "高压参数"=w3278, "电池信息"=w3279) -> (w3276:T4)
                                n1945 = control-ref of="二维码信息"() -> (w3275:refnum<vi>)
                                n1946 = local write "主板数据"(w3276) -> ()
                                }
                                frame #1 {
                                n1947 = control-ref of="主板数据"() -> (w3287:refnum<vi>)
                                }
                                }
                                }
                                frame "从板" {
                                n1948 = stacked-sequence {
                                tunnel: [_ w3299] -> w3288
                                frame #0 {
                                n1949 = control-ref of="从板号"() -> (w3293:refnum<vi>)
                                n1950 = control-ref of="项目信息 2"() -> (w3294:refnum<vi>)
                                n1951 = control-ref of="电池组信息"() -> (w3292:refnum<vi>)
                                n1952 = control-ref of="加热控制参数"() -> (w3295:refnum<vi>)
                                n1953 = control-ref of="一级故障(从板)"() -> (w3296:refnum<vi>)
                                n1954 = control-ref of="二级故障(从板)"() -> (w3297:refnum<vi>)
                                n1955 = control-ref of="三级故障(从板)"() -> (w3298:refnum<vi>)
                                n1956 = control-ref of="均衡参数"() -> (w3291:refnum<vi>)
                                n1957 = local read "从板信息"() -> (w3290:T2)
                                n1958 = Bundle(cluster=w3290, "从板号"=w3293, "项目信息 2"=w3294, "加热控制参数"=w3295, "一级故障(从板)"=w3296, "二级故障(从板)"=w3297, "三级故障(从板)"=w3298, "电池组信息(从板)"=w3292, "均衡参数"=w3291) -> (w3289:T2)
                                n1959 = local write "从板信息"(w3289) -> ()
                                }
                                frame #1 {
                                n1960 = control-ref of="从板信息"() -> (w3299:refnum<vi>)
                                }
                                }
                                }
                              }
                              n1961 = control-ref of="二维码信息 2"() -> (w3262:refnum<vi>)
                              n1962 = control-ref of="结果"() -> (w3269:refnum<vi>)
                              n1963 = control-ref of="从板个数"() -> (w3265:refnum<vi>)
                              n1964 = call "输出数据解析.vi"("主板引用"=w3267, "错误代码"=w3272, "命令序号"=w3271, "输入数组"=w3270, "命令"=w3268, "从板引用"=w3266, "进度引用"=w3269, "板选择"=w3264, "从板个数"=w3265, "二维码信息"=w3263, "从板二维码信息"=w3262) -> ("写入超时"=→"写入超时":bool)  [unwired: 5 in, 3 out]
                            }
                            frame True {
                              n1965 = Index Array(array=w3300, index #1=0 ("索引"), index #2=1 ("索引")) -> (element #1=w3303:u8, element #2=w3304:u8)
                              n1966 = Join Numbers(hi=w3303, lo=w3304) -> ((hi.lo)=w3302:u16)
                              n1967 = Number To Hexadecimal String(2:w3302) -> (0:w3301:string)  [unwired: 1 out]
                              n1968 = control-ref of="结果"() -> (w3309:refnum<vi>)
                              n1969 = Concatenate Strings("0x" ("字符串"), w3301) -> (w3310:string)
                              n1970 = Build Array(w3310) -> (w3311:string[])
                              n1971 = call "表格编辑.vi"("新元素/子数组"=w3311, "活动单元格:单元格背景色"=u32 16740749, "MCListbox引用句柄"=w3309) -> ()  [unwired: 9 out]
                            }
                          }
